vi "inc_forward.vi"(11 "NXT":T1={"Hardware"="NXT", "Flattened String"=""}) -> (3 "NXT2":T1 caption="NXT")   [LabVIEW 2012]
uses:
  <vilib>/NXT/Subs/LVHSConnector.ctl
  <vilib>/NXT/Subs/MotorOutput.ctl
  <vilib>/NXT/Dual Mode Library/Motors/MotorReverse.vi
  <vilib>/NXT/Dual Mode Library/Motors/MotorBrake.vi
  <vilib>/NXT/Dual Mode Library/Waits/Wait_Num(msec).vi
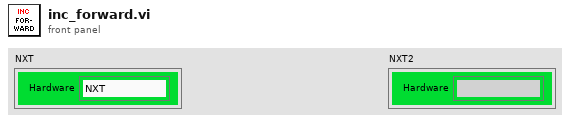
[diagram p1: front panel]
types:
  T1 = typedef "LVHSConnector.ctl" = cluster{"Hardware":string, "Flattened String":string}
  T2 = typedef "MotorOutput.ctl" = u8
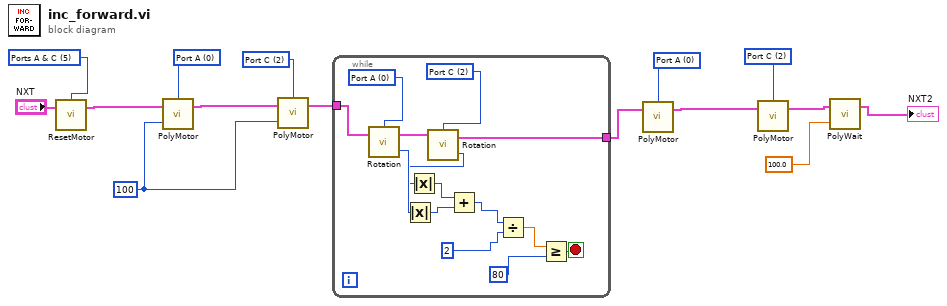
[diagram p0: block diagram]
diagram:
  w8 = T2 2 items=["Port A"=0, "Port B"=1, "Port C"=2, "Ports A & B"=4, "Ports A & C"=5, "Ports B & C"=6, "All Ports"=3] ("Output Port (All Ports)")
  w6 = T2 0 items=["Port A"=0, "Port B"=1, "Port C"=2, "Ports A & B"=4, "Ports A & C"=5, "Ports B & C"=6, "All Ports"=3] ("Output Port (All Ports)")
  w10 = 100
  w12 = T2 2 items=["Port A"=0, "Port B"=1, "Port C"=2, "Ports A & B"=4, "Ports A & C"=5, "Ports B & C"=6, "All Ports"=3] ("Output Port (All Ports)")
  w14 = T2 0 items=["Port A"=0, "Port B"=1, "Port C"=2, "Ports A & B"=4, "Ports A & C"=5, "Ports B & C"=6, "All Ports"=3] ("Output Port (All Ports)")
  w15 = T2 5 items=["Port A"=0, "Port B"=1, "Port C"=2, "Ports A & B"=4, "Ports A & C"=5, "Ports B & C"=6, "All Ports"=3] ("Output Port (All Ports)")
  n1 = call <vilib>:"ResetMotor.vi"("NXT"="NXT", "Port (All Ports)"=w15) -> ("NXT"=w9:T1)  [unwired: 2 in]
  n2 = call-poly <vilib>:"PolyMotor.vi"("Power (75)"=w10, "NXT"=w9, "Output Port (All Ports)"=w14) -> ("NXT"=w13:T1)  [unwired: 1 in]
  n3 = call-poly <vilib>:"PolyMotor.vi"("Power (75)"=w10, "NXT"=w13, "Output Port (All Ports)"=w12) -> ("NXT"=w11:T1)  [unwired: 1 in]
  n4 = while {
    tunnel: w11 -> [w27]
    tunnel: [w26] -> w5
    stop <- w21 stop-if-true
    w25 = T2 2 items=["Port A"=0, "Port B"=1, "Port C"=2, "Ports A & B"=4, "Ports A & C"=5, "Ports B & C"=6, "All Ports"=3] ("Output Port (All Ports)")
    w28 = T2 0 items=["Port A"=0, "Port B"=1, "Port C"=2, "Ports A & B"=4, "Ports A & C"=5, "Ports B & C"=6, "All Ports"=3] ("Output Port (All Ports)")
    n5 = call <vilib>:"Rotation.vi"("NXT"=w27, "Port (Port A)"=w28) -> ("Angle of Rotation"=w17:i32, "NXT"=w29:T1)  [unwired: 1 in]
    n6 = Absolute Value(x=w17) -> (abs(x)=w18:i32)
    n7 = call <vilib>:"Rotation.vi"("NXT"=w29, "Port (Port A)"=w25) -> ("Angle of Rotation"=w16:i32, "NXT"=w26:T1)  [unwired: 1 in]
    n8 = Absolute Value(x=w16) -> (abs(x)=w19:i32)
    n9 = Add(x=w19, y=w18) -> (x+y=w23:i32)
    n10 = Divide(x=w23, y=2) -> (x/y=w22:dbl)
    n11 = Greater Or Equal?(x=w22, y=80) -> (x >= y?=w21:bool)
  }
  n12 = call-poly <vilib>:"PolyMotor.vi"("NXT"=w5, "Port (All Ports)"=w6) -> ("NXT"=w7:T1)  [unwired: 2 in]
  n13 = call-poly <vilib>:"PolyMotor.vi"("NXT"=w7, "Port (All Ports)"=w8) -> ("NXT"=w3:T1)  [unwired: 2 in]
  n14 = call-poly <vilib>:"PolyWait.vi"("Time (100 msec)"=sgl 100.0 ("Time (1 sec)"), "NXT"=w3) -> ("NXT"=→"NXT2":T1)  [unwired: 2 in]
